vi "Add to Definitions.vi"(8 "error in (no error)":errorcluster, 10 "Definition Schema":string, 11 "Name":string) -> (0 "error out":errorcluster)   [LabVIEW 2023, in "JSON Schema Generator.lvlib"]
uses:
  JSON Schema Generator.lvlib
  Defintion FGV Actions.ctl
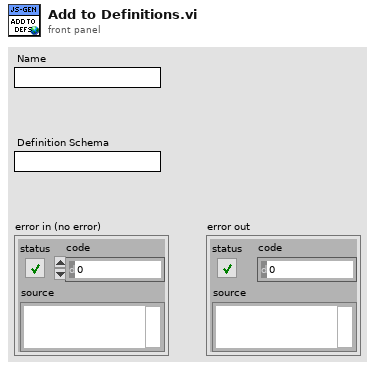
[diagram p1: front panel]
types:
  T1 = typedef "JSON Schema Generator.lvlib/Defintion FGV Actions.ctl" = enum16{"Create Defs", "Update Defs", "Get all Defs", "Get Def"}
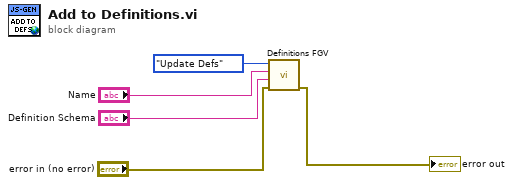
[diagram p0: block diagram]
diagram:
  n1 = call "Definitions FGV.vi"("error in (no error)"="error in (no error)", "Defintion Schema In"="Definition Schema", "Definition Name"="Name", "Action"=Defintion_FGV_Actions."Update Defs") -> ("error out"=→"error out":errorcluster)  [unwired: 5 in, 2 out]
